vi "Test queue of shared variable.vi"() -> ()   [LabVIEW 2013]
panel:
  out "element":string
  out "Received Data":string
  in  "stop 2":bool
  in  "stop":bool
  in  "Boolean":bool
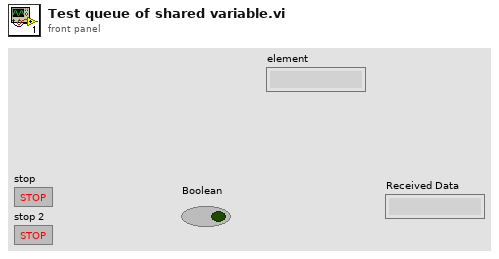
[diagram p1: front panel]
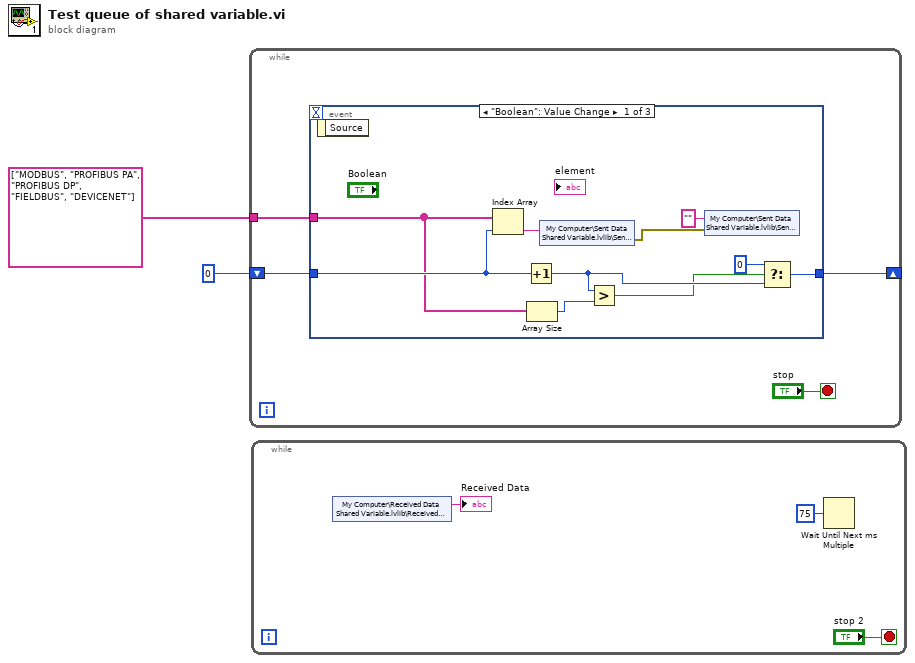
[diagram p0: block diagram]
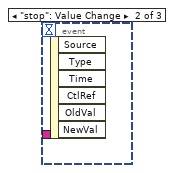
[diagram p2: hidden frame]
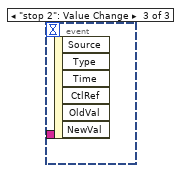
[diagram p3: hidden frame]
diagram:
  n1 = while {
    tunnel: string[] ["MODBUS", "PROFIBUS PA", "PROFIBUS DP", "FIELDBUS", "DEVICENET"] -> [w5]
    shift-right: [w3] -> _
    shift-left: 0 ("index") -> [w4]
    stop <- "stop" stop-if-true
    n2 = event shown="[0] \"Boolean\": Value Change" {
      selector: _ -> [_ _ _]
      dyn-events: _ -> [_ _ _]
      timeout: _ -> [_ _ _]
      tunnel: w5 -> [w13 _ _]
      tunnel: w4 -> [w16 _ _]
      tunnel: [w10 _ _] -> w3
      event "Boolean": Value Change {
        n3 = event-data() -> ()  [unwired: 1 in, 1 out]
        n4 = Index Array(array=w13, index=w16) -> (element=w15:string)
        n5 = Increment(x=w16) -> (x+1=w12:i32)
        n6 = Array Size(array=w13) -> (size(s)=w14:i32)
        n7 = shared-variable "My Computer\\Sent Data Shared Variable.lvlib\\Sent Data"(w15) -> (error out=w8:errorcluster)  [unwired: 1 in]
        n8 = Greater?(x=w12, y=w14) -> (0:w11:bool)
        n9 = shared-variable "My Computer\\Sent Data Shared Variable.lvlib\\Sent Data"("" ("Sent Data"), error in=w8) -> ()  [unwired: 1 out]
        n10 = Select(t=0, s=w11, f=w12) -> (s? t:f=w10:i32)
      }
      event "stop": Value Change {
        n11 = event-data() -> ()  [unwired: 1 in, 6 out]
      }
      event "stop 2": Value Change {
        n12 = event-data() -> ()  [unwired: 1 in, 6 out]
      }
    }
  }
  n13 = while {
    stop <- "stop 2" stop-if-true
    n14 = shared-variable "My Computer\\Received Data Shared Variable.lvlib\\Received Data"() -> (→"Received Data":string)  [unwired: 1 in, 1 out]
    n15 = Wait Until Next ms Multiple(millisecond multiple=u32 75) -> ()  [unwired: 1 out]
  }
